vi "Display Console View.vi"(8 "error in (no error)":errorcluster, 11 "View Model":T1) -> (0 "error out":errorcluster)   [LabVIEW 2017]
doc: "The interface where a user receives status updates from the ATM Controller.\n[Covers: UI3]"
uses:
  View Model/Controls/View Model.ctl
  View Model/Controls/Shared Model.ctl
  Error Handler/Controls/Error Model.ctl
  Error Handler/Controls/Error Data.ctl
  Error Handler/Controls/Error Type.ctl
  Error Handler/Controls/Error Source.ctl
  Configuration/Controls/Config Model.ctl
  Configuration/Controls/Config CMD.ctl
  Configuration/Controls/Config Command.ctl
  Controller/Controls/Controller Model.ctl
  Controller/Controls/Controller Overhead.ctl
  Controller/Controls/Controller Transaction.ctl
  Controller/Controls/Controller State.ctl
  Configuration/Controls/Config Data Record.ctl
  Controls/Display Console - References.ctl
panel:
  out "Card Read":bool
  out "Message Screen":string
  out "Current Transaction":string
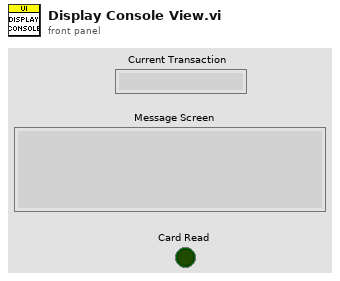
[diagram p1: front panel]
types:
  T1 = typedef "View Model.ctl" = cluster{"Shared Model":T2, "Error Model":T3, "Config Model":T4, "Controller Model":T5}
  T2 = typedef "Shared Model.ctl" = cluster{"Stop":refnum<user-event>, "Stop DVR":refnum<data-value>}
  T3 = typedef "Error Model.ctl" = cluster{"Error":refnum<user-event>}
  T4 = typedef "Config Model.ctl" = cluster{"Config CMD":refnum<user-event>}
  T5 = typedef "Controller Model.ctl" = cluster{"Deposit Received":refnum<user-event>, "Funds Dispensed":refnum<user-event>, "Overhead DVR":refnum<data-value>, "Entered Num":refnum<user-event>, "Card Read":refnum<user-event>, "Transaction":refnum<user-event>}
  T6 = typedef "Display Console - References.ctl" = cluster{"Card Read":refnum<vi>, "Transaction":refnum<vi>, "Message ":refnum<vi>}
  T7 = typedef "Controller State.ctl" = enum16{"Idle", "Initial", "Login", "Balance Inquiry", "Deposit", "Withdrawal", "Fast Cash", "Terminate"}
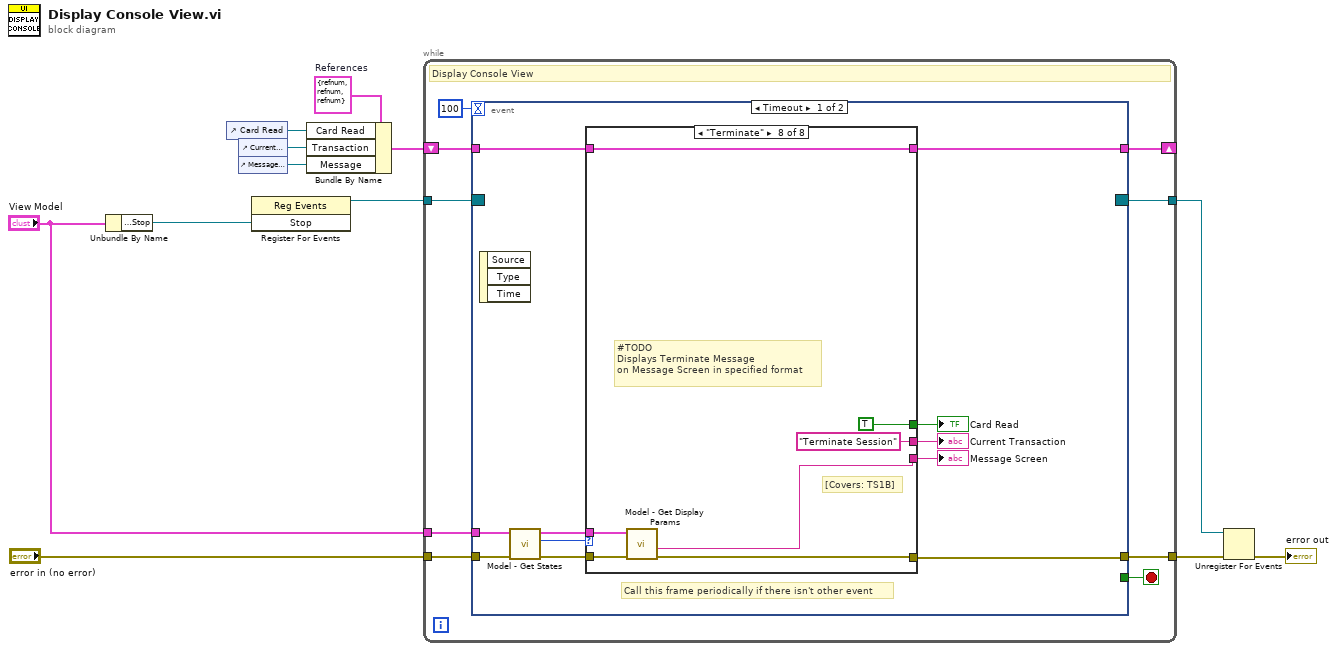
[diagram p0: block diagram]
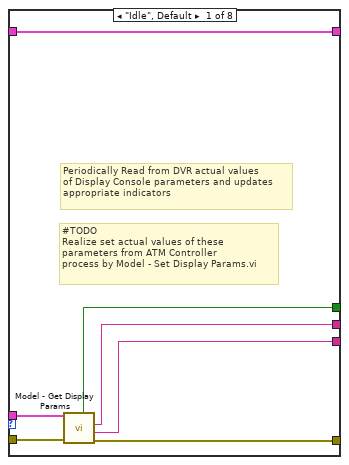
[diagram p2: hidden frame]
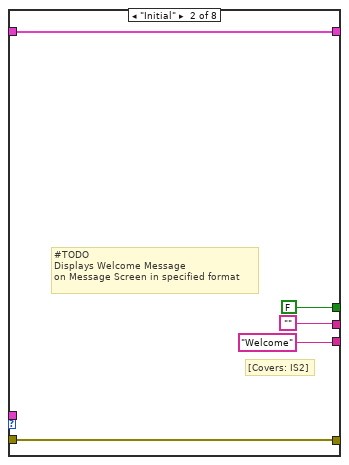
[diagram p3: hidden frame]
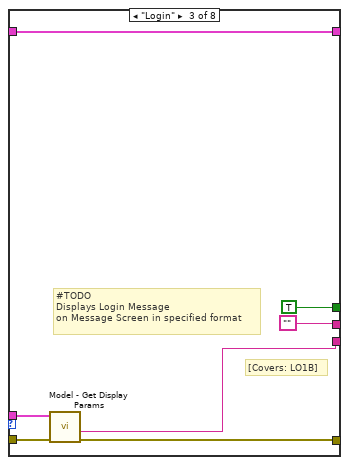
[diagram p4: hidden frame]
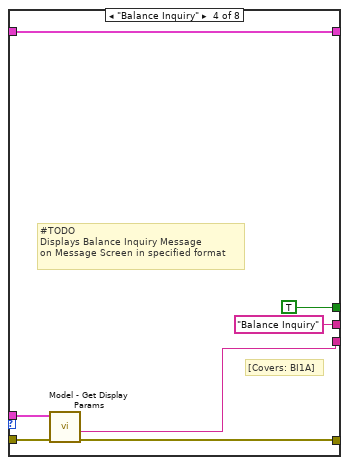
[diagram p5: hidden frame]
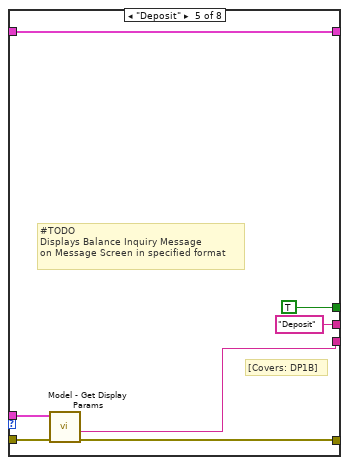
[diagram p6: hidden frame]
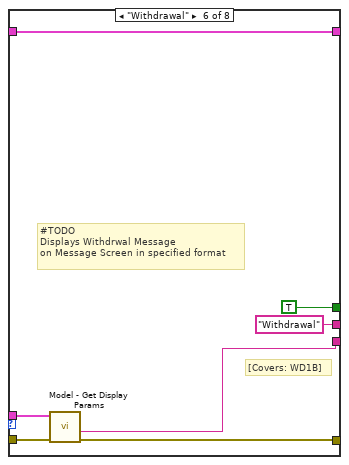
[diagram p7: hidden frame]
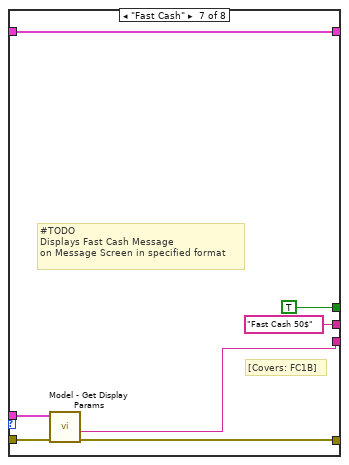
[diagram p8: hidden frame]
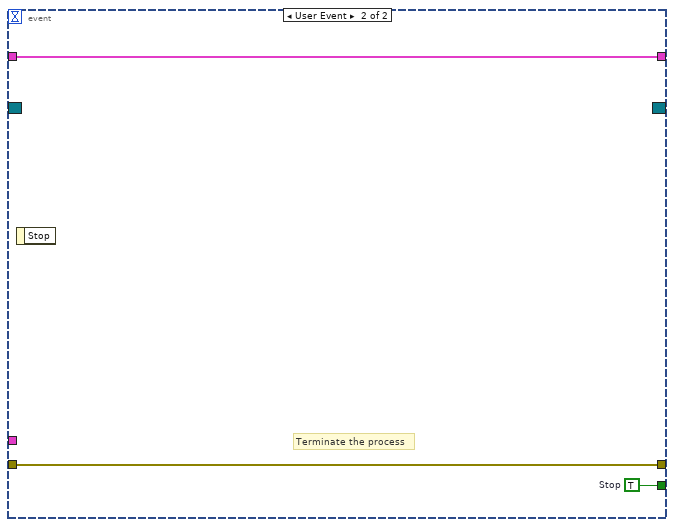
[diagram p9: hidden frame]
diagram:
  w6 = T6 {"Card Read"=refnum, "Transaction"=refnum, "Message "=refnum}  # References
  n1 = Unbundle By Name("View Model") -> ("Shared Model.Stop"=w12:refnum<user-event>)
  n2 = control-ref of="Card Read"() -> (w5:refnum<vi>)
  n3 = control-ref of="Current Transaction"() -> (w4:refnum<vi>)
  n4 = control-ref of="Message Screen"() -> (w3:refnum<vi>)
  n5 = register-events(w12) -> (reference out=w11:refnum<event-registration>)  [unwired: 2 in, 1 out]
  n6 = Bundle By Name(cluster=w6, "Card Read"=w5, "Transaction"=w4, "Message"=w3) -> (w2:T6)
  n7 = while {
    tunnel: w11 -> [w21]
    tunnel: [w20] -> w10
    tunnel: "error in (no error)" -> [w19]
    tunnel: [w18] -> w8
    tunnel: "View Model" -> [w15]
    shift-right: [w13] -> _
    shift-left: w2 -> [w14]
    stop <- w16 stop-if-true
    # "Display Console View"
    n8 = event shown="[0] Timeout" {
      selector: w21 -> [_ _]
      dyn-events: [_ _] -> w20
      timeout: 100 -> [_ _]
      tunnel: w19 -> [w32 w89]
      tunnel: [w26 w89] -> w18
      tunnel: [_ w88] -> w16
      tunnel: w15 -> [w31 _]
      tunnel: w14 -> [w29 w87]
      tunnel: [w25 w87] -> w13
      event Timeout {
        # "Call this frame periodically if there isn't other event"
        n9 = event-data() -> ()  [unwired: 1 in, 3 out]
        n10 = call "Model - Get States.vi"("error in (no error)"=w32, "View Model"=w31) -> ("error out"=w27:errorcluster, "Current State"=w30:T7, "View Model"=w28:T1)  [unwired: 6 in, 1 out]
        n11 = case shown="\"Terminate\"" w30 {
          tunnel: w29 -> [w36 w44 w51 w58 w65 w72 w79 w86]
          tunnel: w28 -> [w39 _ w48 w56 w63 w70 w77 w84]
          tunnel: w27 -> [w38 w43 w47 w55 w62 w69 w76 w83]
          tunnel: [w37 w43 w46 w54 w61 w68 w75 w82] -> w26
          tunnel: [w36 w44 w51 w58 w65 w72 w79 w86] -> w25
          tunnel: [w35 FALSE ("Card Read") TRUE ("Card Read") TRUE ("Card Read") TRUE ("Card Read") TRUE ("Card Read") TRUE ("Card Read") TRUE ("Card Read")] -> w24
          tunnel: [w34 "" "" "Balance Inquiry" ("Current Transaction") "Deposit" ("Current Transaction") "Withdrawal" ("Current Transaction") "Fast Cash 50$" ("Current Transaction") "Terminate Session" ("Current Transaction")] -> w23
          tunnel: [w33 "Welcome" ("Message Screen") w45 w53 w60 w67 w74 w81] -> w22
          frame "Idle", Default {
            # "#TODO\nRealize set actual values of these\nparameters from ATM Controller\nprocess by Model - Set Display Params.vi"
            # "Periodically Read from DVR actual values\nof Display Console parameters and updates\nappropriate indicators"
            n12 = call "Model - Get Display Params.vi"("error in (no error)"=w38, "View Model"=w39) -> ("error out"=w37:errorcluster, "Message"=w33:string, "Current Transaction"=w34:string, "Card Read"=w35:bool)  [unwired: 5 in, 1 out]
          }
          frame "Initial" {
            # "[Covers: IS2]"
            # "#TODO\nDisplays Welcome Message\non Message Screen in specified format"
          }
          frame "Login" {
            # "[Covers: LO1B]"
            # "#TODO\nDisplays Login Message\non Message Screen in specified format"
            n13 = call "Model - Get Display Params.vi"("error in (no error)"=w47, "View Model"=w48) -> ("error out"=w46:errorcluster, "Message"=w45:string)  [unwired: 5 in, 3 out]
          }
          frame "Balance Inquiry" {
            # "[Covers: BI1A]"
            # "#TODO\nDisplays Balance Inquiry Message\non Message Screen in specified format"
            n14 = call "Model - Get Display Params.vi"("error in (no error)"=w55, "View Model"=w56) -> ("error out"=w54:errorcluster, "Message"=w53:string)  [unwired: 5 in, 3 out]
          }
          frame "Deposit" {
            # "[Covers: DP1B]"
            # "#TODO\nDisplays Balance Inquiry Message\non Message Screen in specified format"
            n15 = call "Model - Get Display Params.vi"("error in (no error)"=w62, "View Model"=w63) -> ("error out"=w61:errorcluster, "Message"=w60:string)  [unwired: 5 in, 3 out]
          }
          frame "Withdrawal" {
            # "[Covers: WD1B]"
            # "#TODO\nDisplays Withdrwal Message\non Message Screen in specified format"
            n16 = call "Model - Get Display Params.vi"("error in (no error)"=w69, "View Model"=w70) -> ("error out"=w68:errorcluster, "Message"=w67:string)  [unwired: 5 in, 3 out]
          }
          frame "Fast Cash" {
            # "[Covers: FC1B]"
            # "#TODO\nDisplays Fast Cash Message\non Message Screen in specified format"
            n17 = call "Model - Get Display Params.vi"("error in (no error)"=w76, "View Model"=w77) -> ("error out"=w75:errorcluster, "Message"=w74:string)  [unwired: 5 in, 3 out]
          }
          frame "Terminate" {
            # "[Covers: TS1B]"
            # "#TODO\nDisplays Terminate Message\non Message Screen in specified format"
            n18 = call "Model - Get Display Params.vi"("error in (no error)"=w83, "View Model"=w84) -> ("error out"=w82:errorcluster, "Message"=w81:string)  [unwired: 5 in, 3 out]
          }
        }
        "Current Transaction" <- w23
        "Message Screen" <- w22
        "Card Read" <- w24
      }
      event User Event {
        w88 = TRUE  # Stop
        # "Terminate the process"
        n19 = event-data() -> ()  [unwired: 1 in, 1 out]
      }
    }
  }
  n20 = Unregister For Events(event registration refnum=w10, error in=w8) -> (error out=→"error out":errorcluster)
